vi "dE_dNet.vi"(10 "Target":fxp<+/-,64,32>[](array[numeric]), 11 "Curren Layer OP":fxp<+/-,64,32>[](array[numeric])) -> (3 "dE/dNet":fxp<+/-,64,32>[](array[numeric]))   [LabVIEW 2014]
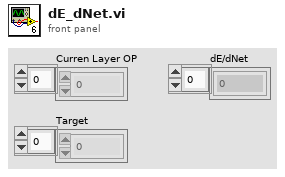
[diagram p1: front panel]
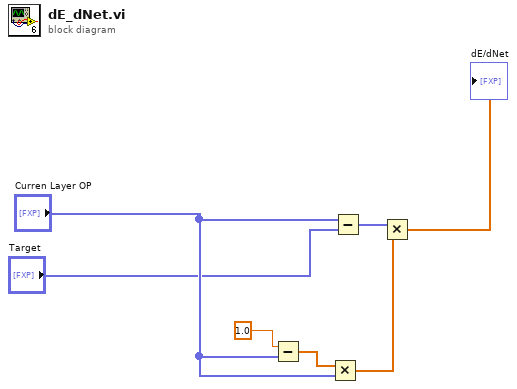
[diagram p0: block diagram]
diagram:
  n1 = Subtract(x=1.0, y="Curren Layer OP") -> (x-y=w6:dbl[])
  n2 = Multiply(x=w6, y="Curren Layer OP") -> (x*y=w1:dbl[])
  n3 = Subtract(x="Curren Layer OP", y="Target") -> (x-y=w3:fxp<+/-,64,33>[])
  n4 = Multiply(x=w3, y=w1) -> (x*y=→"dE/dNet":dbl[])
